vi "cmc-function-gen-witharea.vi"() -> ()   [LabVIEW 2010]
panel:
  out "approximate area under curve":dbl
  out "XY Graph":cluster{"Y":dbl[], "Y":dbl[]}[](graph)
  out "f(x) Array":dbl[](array[numeric])
  out "x Array":dbl[](array[numeric])
  in  "# of divisions":u32
  in  "end x = 'b'":dbl
  in  "Start x = 'a'":dbl
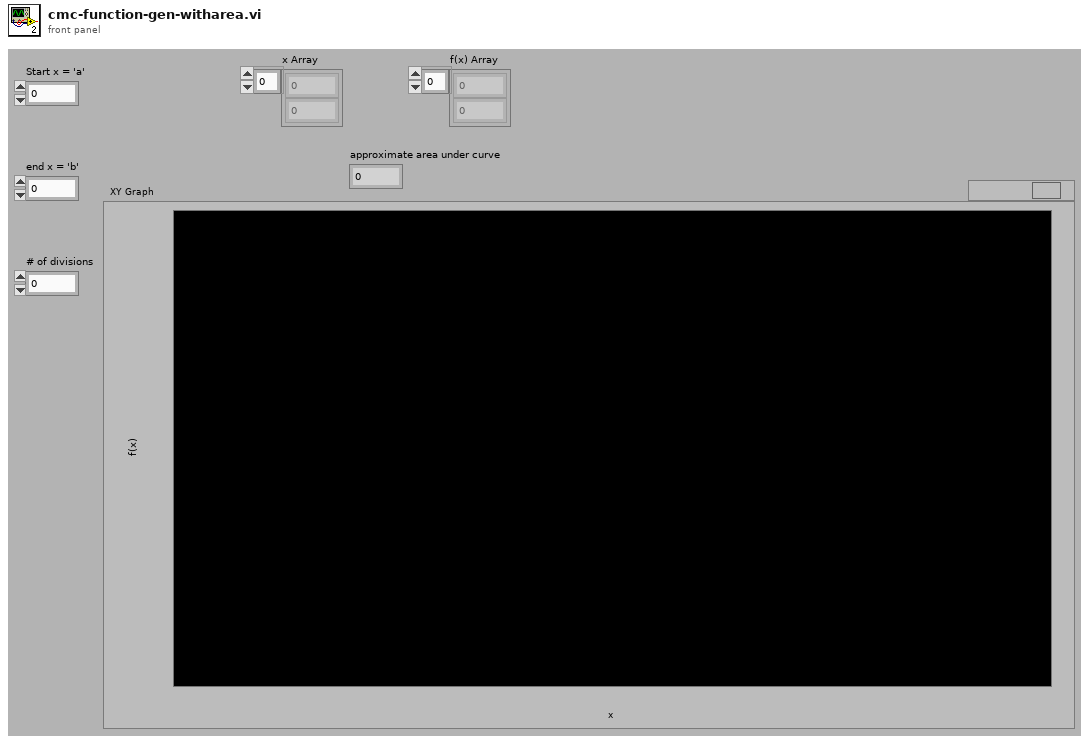
[diagram p1: front panel]
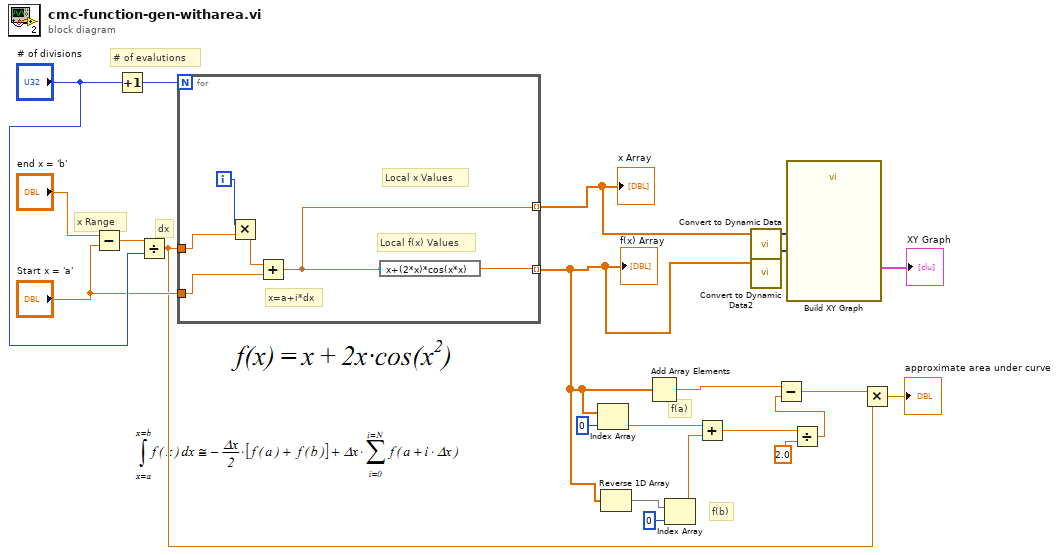
[diagram p0: block diagram]
diagram:
  # "f(b)"
  # "f(a)"
  # "dx"
  # "x Range"
  # "# of evalutions"
  n1 = Subtract(x="end x = 'b'", y="Start x = 'a'") -> (x-y=w21:dbl)
  n2 = Increment(x="# of divisions") -> (x+1=w22:u32)
  n3 = Divide(x=w21, y="# of divisions") -> (x/y=w9:dbl)
  n4 = for {
    N: w22 -> [_]
    tunnel: w9 -> [w27]
    tunnel: "Start x = 'a'" -> [w26]
    tunnel: [w24] -> w16 mode=indexing
    tunnel: [w23] -> w8 mode=indexing
    i -> [w28]
    # "Local f(x) Values"
    # "x=a+i*dx"
    # "Local x Values"
    n5 = Multiply(x=w28, y=w27) -> (x*y=w25:dbl)
    n6 = Add(x=w25, y=w26) -> (x+y=w24:dbl)
    n7 = expression code="x+(2*x)*cos(x*x)"(w24) -> (w23:dbl)
  }
  "x Array" <- w16
  "f(x) Array" <- w8
  n8 = Index Array(array=w8, index=0) -> (element=w10:dbl)
  n9 = Reverse 1D Array(array=w8) -> (reversed array=w6:dbl[])
  n10 = Add Array Elements(numeric array=w8) -> (sum=w13:dbl)
  n11 = Index Array(array=w6, index=0) -> (element=w5:dbl)
  n12 = Add(x=w10, y=w5) -> (x+y=w3:dbl)
  n13 = call "Convert to Dynamic Data"("Array"=w16) -> ("Dynamic Data Type"=w15:dynamicdata)  [unwired: 3 in]
  n14 = call "Convert to Dynamic Data2"("Array"=w8) -> ("Dynamic Data Type"=w14:dynamicdata)  [unwired: 3 in]
  n15 = call "Build XY Graph"("Y Input"=w14, "X Input"=w15) -> ("XY Graph"=→"XY Graph":cluster{"Y":dbl[], "Y":dbl[]}[])  [unwired: 3 in, 6 out]
  n16 = Divide(x=w3, y=2.0) -> (x/y=w2:dbl)
  n17 = Subtract(x=w13, y=w2) -> (x-y=w12:dbl)
  n18 = Multiply(x=w12, y=w9) -> (x*y=→"approximate area under curve":dbl)
